vi "Initialize.vi"(8 "error in (no error)":errorcluster, 11 "Software Lock-in in":refnum<class "Lock-in Detector.lvclass">) -> (0 "error out":errorcluster, 3 "Software Lock-in out":refnum<class "Lock-in Detector.lvclass">, 5 "found":bool=TRUE)   [LabVIEW 2020, in "Lock-in Detector.lvclass"]
uses:
  Lock-in Detector.lvclass
  Lock-in Detector.lvclass/Lock-in Detector.ctl
  Read Sample rate.vi
  Read Time constant.vi
  Write Reference phase.vi
  Write Reference frequency.vi
  Write Reference amplitude.vi
  Write Decimation factor.vi
  Write Decimation position.vi
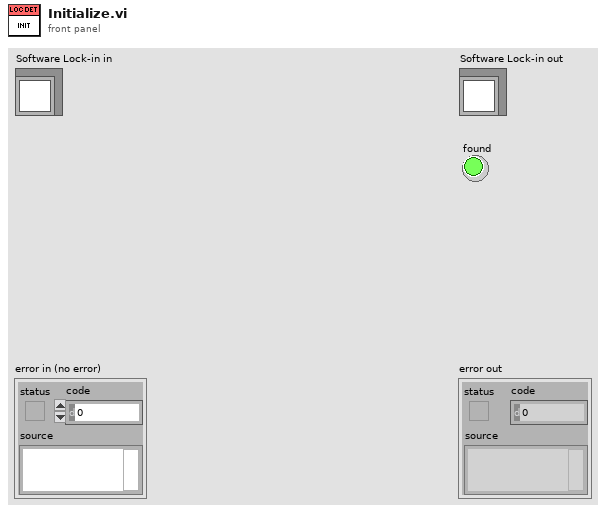
[diagram p1: front panel]
types:
  T1 = typedef "Lockin Parameters.ctl" = cluster{"Frequency":dbl, "Phase":dbl, "Syncronous":bool, "Points per sine wave":i32, "DDS":bool, "Frequency word":u32, "Phase word":u32, "DDS modulus":i64, "DDS clock":dbl}
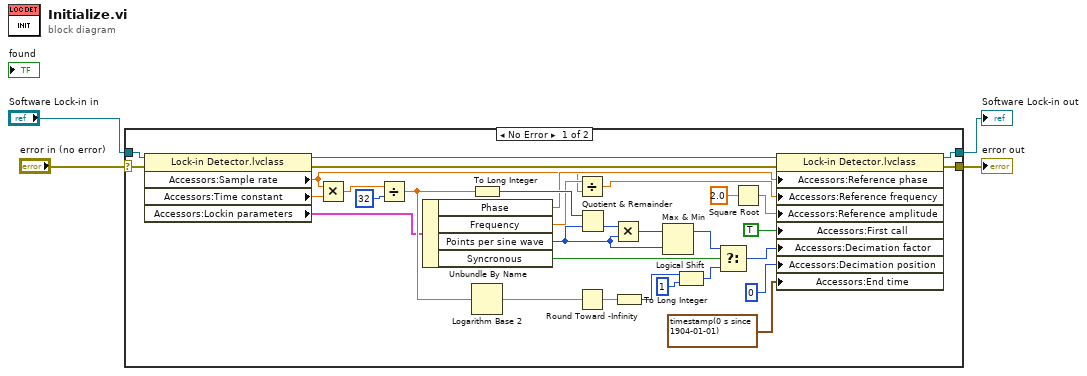
[diagram p0: block diagram]
diagram:
  n1 = case shown="No Error" "error in (no error)" {
    selector: "error in (no error)" -> [w35 w38]
    tunnel: [w34 w38] -> w3
    tunnel: [w36 w37] -> w1
    tunnel: "Software Lock-in in" -> [w6 w37]
    frame No Error {
      n2 = property class="Lock-in Detector.lvclass"(reference=w6, error in=w35) -> (reference out=w7:refnum<class "Lock-in Detector.lvclass">, error out=w17:errorcluster, "Accessors:Sample rate"=w8:dbl, "Accessors:Time constant"=w9:dbl, "Accessors:Lockin parameters"=w10:T1)
      n3 = Multiply(x=w8, y=w9) -> (x*y=w32:dbl)
      n4 = Divide(x=w32, y=32) -> (x/y=w24:dbl)
      n5 = Unbundle By Name(w10) -> ("Phase"=w16:dbl, "Frequency"=w20:dbl, "Points per sine wave"=w19:i32, "Syncronous"=w18:bool)
      n6 = To Long Integer(number=w24) -> (32bit integer=w25:i32)
      n7 = Logarithm Base 2(1:w24) -> (0:w30:dbl)
      n8 = Divide(x=w20, y=w8) -> (x/y=w15:dbl)
      n9 = Round Toward -Infinity(1:w30) -> (0:w29:dbl)
      n10 = Quotient & Remainder(x=w25, y=w19) -> (floor(x/y)=w23:i32)  [unwired: 1 out]
      n11 = Multiply(x=w23, y=w19) -> (x*y=w22:i32)
      n12 = To Long Integer(number=w29) -> (32bit integer=w27:i32)
      n13 = Max & Min(x=w22, y=w19) -> (max(x,y)=w21:i32)  [unwired: 1 out]
      n14 = Logical Shift(y=w27, x=1) -> (x << y=w26:i32)
      n15 = Select(t=w21, s=w18, f=w26) -> (s? t:f=w12:i32)
      n16 = Square Root(x=2.0 ("1/x")) -> (sqrt(x)=w14:dbl)
      n17 = property class="Lock-in Detector.lvclass"(reference=w7, error in=w17, "Accessors:Reference phase"=w16, "Accessors:Reference frequency"=w15, "Accessors:Reference amplitude"=w14, "Accessors:First call"=TRUE ("First call"), "Accessors:Decimation factor"=w12, "Accessors:Decimation position"=0 ("Decimation position"), "Accessors:End time"=timestamp(0 s since 1904-01-01) ("End time")) -> (reference out=w36:refnum<class "Lock-in Detector.lvclass">, error out=w34:errorcluster)
    }
    frame Error {
    }
  }
  "error out" <- w3
  "Software Lock-in out" <- w1
